vi "Add Source File.vi"(8 "error in (no error)":errorcluster, 10 "Source File":path, 11 "Session in":refnum<class "Session.lvclass">) -> (0 "error out":errorcluster, 3 "Session out":refnum<class "Session.lvclass">)   [LabVIEW 2020, in "Save for Previous Version.lvlib" / "Session.lvclass"]
uses:
  Session.lvclass
  Session.lvclass/Session.ctl
  File/File.lvclass/File.lvclass
  Save for Previous Version.lvlib
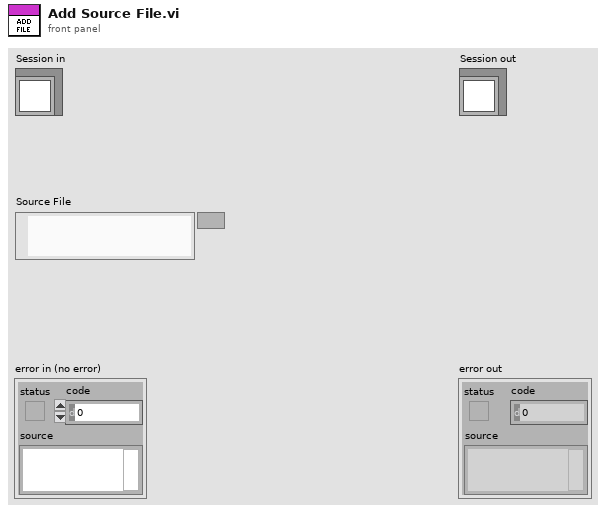
[diagram p1: front panel]
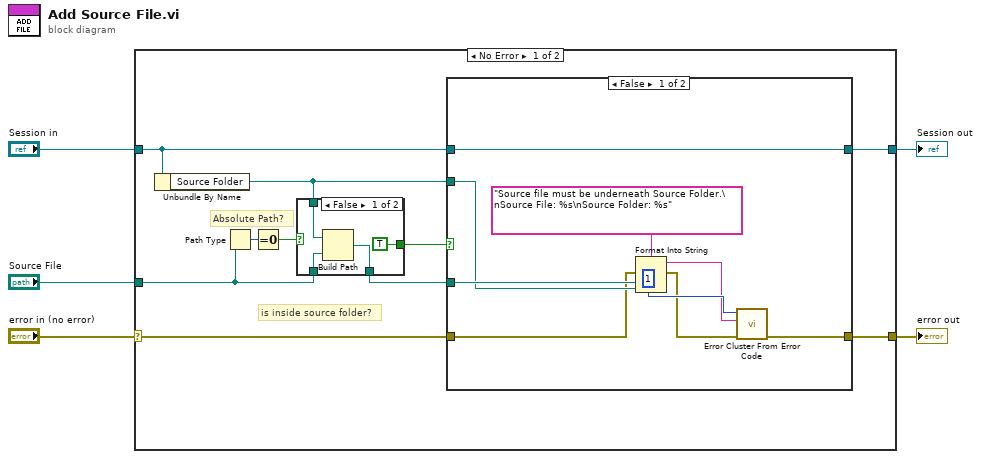
[diagram p0: block diagram]
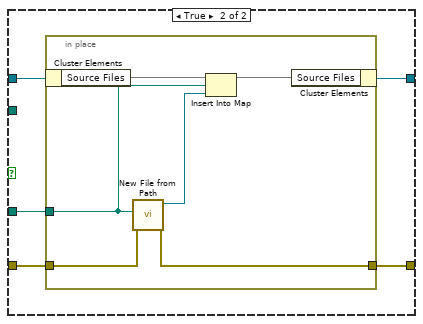
[diagram p2: hidden frame]
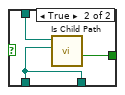
[diagram p3: hidden frame]
diagram:
  n1 = case shown="No Error" "error in (no error)" {
    selector: "error in (no error)" -> [w14 w44]
    tunnel: [w13 w44] -> w4
    tunnel: [w15 w43] -> w2
    tunnel: "Session in" -> [w9 w43]
    tunnel: "Source File" -> [w10 _]
    frame No Error {
      # "Absolute Path?"
      # "is inside source folder?"
      n2 = Unbundle By Name(w9) -> ("Source Folder"=w8:path)
      n3 = Path Type(1:w10) -> (0:w11:i16)
      n4 = Equal To 0?(x=w11) -> (x = 0?=w12:bool)
      n5 = case shown="False" w12 {
        tunnel: w8 -> [w38 w42]
        tunnel: [TRUE ("is Child Path") w41] -> w6
        tunnel: w10 -> [w39 w40]
        tunnel: [w37 w40] -> w7
        frame False {
          n6 = Build Path(base path=w38, name or relative path=w39) -> (appended path=w37:path)
        }
        frame True {
          n7 = call "Is Child Path.vi"("File"=w40, "Base Folder"=w42) -> ("is Child Path"=w41:bool)  [unwired: 8 in, 1 out]
        }
      }
      n8 = case shown="False" w6 {
        tunnel: w9 -> [w24 w29]
        tunnel: w7 -> [w20 w28]
        tunnel: [w24 w27] -> w15
        tunnel: [w23 w26] -> w13
        tunnel: w14 -> [w16 w25]
        tunnel: w8 -> [w19 _]
        frame False {
          n9 = Format Into String(format string="Source file must be underneath Source Folder.\nSource File: %s\nSource Folder: %s", error in=w16, w20, w19) -> (resulting string=w18:string, error out=w17:errorcluster)  [unwired: 1 in]
          n10 = call <vilib>:"Error Cluster From Error Code.vi"("error in (no error)"=w17, "error message (\"\")"=w18, "error code (0)"=1) -> ("error out"=w23:errorcluster)  [unwired: 6 in]
        }
        frame True {
          n11 = in-place {
            in-place-border: w28 -> [w32]
            in-place-border: [w35] -> w26
            in-place-border: w25 -> [w34]
            n12 = in-place-cluster #1(w29) -> ("Source Files"=w33:map{path, refnum<class "File.lvclass">})
            n13 = call "New File from Path.vi"("error in (no error)"=w34, "Path"=w32) -> ("error out"=w35:errorcluster, "File out"=w30:refnum<class "File.lvclass">)  [unwired: 8 in]
            n14 = Insert Into Map(map in=w33, key=w32, value=w30) -> (map out=w31:map{path, refnum<class "File.lvclass">})  [unwired: 2 out]
            n15 = in-place-cluster #1("Source Files"=w31) -> (w27:refnum<class "Session.lvclass">)
          }
        }
      }
    }
    frame Error {
    }
  }
  "error out" <- w4
  "Session out" <- w2
